vi "websocket (un)mask data.vi"(10 "mask key":u32, 11 "masked data":string) -> (3 "unmasked data":string)   [LabVIEW 2016, in "websocket core.lvlib"]
uses:
  websocket core.lvlib
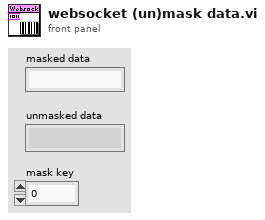
[diagram p1: front panel]
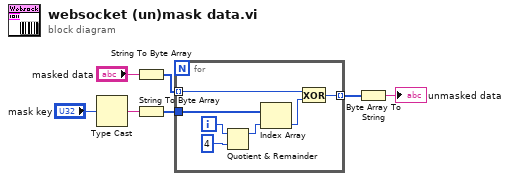
[diagram p0: block diagram]
diagram:
  n1 = Type Cast(x="mask key") -> (*(type *) &x=w4:string)  [unwired: 1 in]
  n2 = String To Byte Array(string="masked data") -> (unsigned byte array=w2:u8[])
  n3 = String To Byte Array(string=w4) -> (unsigned byte array=w5:u8[])
  n4 = for {
    tunnel: w2 -> [w12] mode=indexing
    tunnel: w5 -> [w13]
    tunnel: [w10] -> w6 mode=indexing
    i -> [w14]
    n5 = Quotient & Remainder(x=w14, y=4) -> (x-y*floor(x/y)=w8:i32)  [unwired: 1 out]
    n6 = Index Array(array=w13, index=w8) -> (element=w11:u8)
    n7 = Exclusive Or(1:w11, 2:w12) -> (0:w10:u8)
  }
  n8 = Byte Array To String(unsigned byte array=w6) -> (string=→"unmasked data":string)
